vi "BRig_dataCurrent_DAB_T_Reward_R.vi"() -> (2 "output_DAB_T_Reward_R":i32)   [LabVIEW 2014]
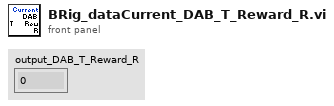
[diagram p1: front panel]
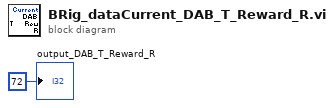
[diagram p0: block diagram]
diagram:
  "output_DAB_T_Reward_R" <- 72 ("output_iBlock")
